vi "Teleop.vi"(10 "Match Info":T1={"Autonomous Elapsed Seconds"=0.0, "TeleOp Elapsed Seconds"=0.0, "Disabled Elapsed Seconds"=0.0, "Visited Autonomous"=FALSE, "Visited TeleOp"=FALSE, "Visited Disabled"=FALSE, "Autonomous Settings"={"Autonomous Style"=enum."Independent", "VI Refnum"=refnum}}, 11 "Call Context":T2) -> ()   [LabVIEW 2018]
doc: "This VI is called for each enabled TeleOp packet received from the DS. It is typically used to read from joysticks and other inputs and update I/O or setpoints for timed control loops. It should complete and return within 20 milliseconds or risk missing DS packets."
uses:
  <vilib>/Rock Robotics/WPI/DriverStation/WPI_DriverStationDerivedRobotMode.ctl
  <vilib>/Rock Robotics/WPI/DriverStation/WPI_DriverStationMatch Info.ctl
  <vilib>/Rock Robotics/WPI/Utilities/WPI_GetSetVariantRefNum.vi
  <vilib>/Rock Robotics/Network Tables/NT Write Boolean Array.vi
  <vilib>/Rock Robotics/Network Tables/NT Write Numeric Array.vi
  <vilib>/Rock Robotics/WPI/Ultrasonic/WPI_SonarMB1010AnalogRefNum Registry Get.vi
  <vilib>/Rock Robotics/WPI/Ultrasonic/WPI_SonarMB1010AnalogGetRange.vi
  Framework/Robot Global Data.vi
panel:
  out "Safe to drive Back (UnZucced)":bool
  out "Zucced?":bool
  in  "Sensor Margin of Error":dbl=2.0
  in  "Acceptable Hab Distance":dbl=12.0
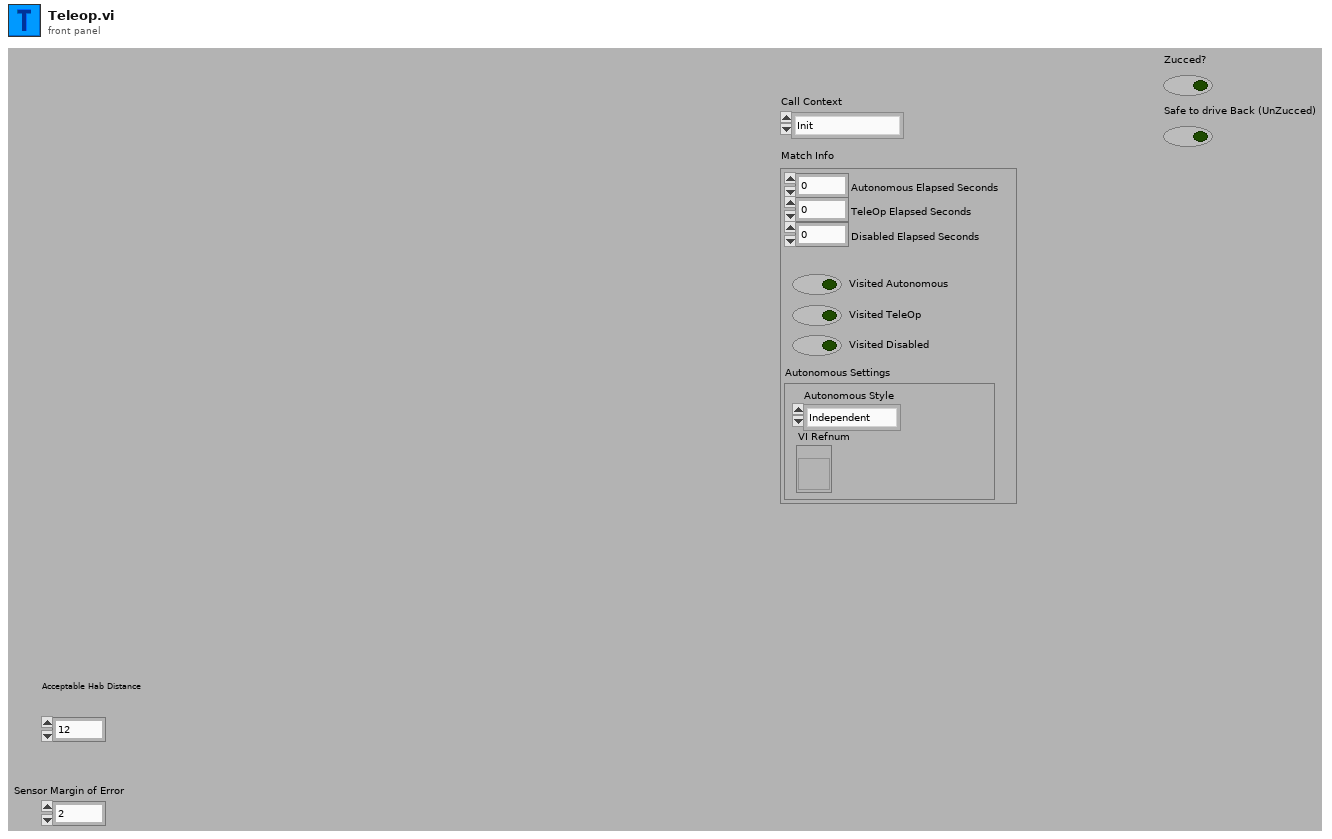
[diagram p1: front panel]
types:
  T1 = typedef "WPI_DriverStationMatch Info.ctl" = cluster{"Autonomous Elapsed Seconds":dbl, "TeleOp Elapsed Seconds":dbl, "Disabled Elapsed Seconds":dbl, "Visited Autonomous":bool, "Visited TeleOp":bool, "Visited Disabled":bool, "Autonomous Settings":cluster{"Autonomous Style":enum16{"Iterative", "Independent"}, "VI Refnum":refnum<vi>}}
  T2 = typedef "WPI_DriverStationDerivedRobotMode.ctl" = enum16{"Init", "Execute", "Stop"}
  T3 = typedef "WPI_JoystickDevRef.ctl" = cluster{"Device":T4}
  T4 = typedef "WPI_JoystickDeviceEnum.ctl" = enum16{"USB 0", "USB 1", "USB 2", "USB 3", "USB 4", "USB 5"}
  T5 = typedef "WPI_SonarMB1010AnalogDeviceRef.ctl" = cluster{"AIDeviceRef":T6, "Scaling factor (V/in)":dbl, "Average Bits":u8}
  T6 = typedef "WPI_AnalogChannelDevRef.ctl" = cluster{"DevStatus":errorcluster, "Analog Channel":T7}
  T7 = typedef "FPGA_AIChannel.ctl" = enum8{"AI 0", "AI 1", "AI 2", "AI 3", "AI MXP 0", "AI MXP 1", "AI MXP 2", "AI MXP 3", "Invalid"}
  T8 = typedef "WPI_ServoDeviceRef.ctl" = cluster{"DeviceStatus":errorcluster, "PWM Channel":T9, "DeadBand":T10}
  T9 = typedef "FPGA_DIOPWMChannel.ctl" = enum8{"PWM 0", "PWM 1", "PWM 2", "PWM 3", "PWM 4", "PWM 5", "PWM 6", "PWM 7", "PWM 8", "PWM 9", "PWM MXP 0", "PWM MXP 1", "PWM MXP 2", "PWM MXP 3", "PWM MXP 4", "PWM MXP 5", "PWM MXP 6", "PWM MXP 7", "PWM MXP 8", "PWM MXP 9", "Invalid"}
  T10 = typedef "WPI_PWMDeadband.ctl" = cluster{"Name":string, "maxPositivePwm":i32, "minPositivePwm":i32, "centerPwm":i32, "maxNegativePwm":i32, "minNegativePwm":i32, "angularRange":u16}
  T11 = typedef "WPI_MotorControlDeviceRef.ctl" = cluster{"DeviceStatus":errorcluster, "Type":T12, "PWM":cluster{"PWM Channel":T9, "DeadBand":T10}, "CAN":cluster{"Device Number":u8, "SetOutput VI Ref":variant, "GetOutput VI Ref":variant, "Enable VI Ref":variant, "Disable VI Ref":variant, "Data":variant}, "Invert":bool, "DIO PWM":cluster{"PWM \"Enable\" Channel":T9, "DIOChannel":T13, "PWM Rate":dbl}}
  T12 = typedef "WPI_MotorControlType.ctl" = enum16{"PWM", "CAN", "DIO PWM"}
  T13 = typedef "FPGA_DIOChannel.ctl" = enum8{"DIO 0", "DIO 1", "DIO 2", "DIO 3", "DIO 4", "DIO 5", "DIO 6", "DIO 7", "DIO 8", "DIO 9", "DIO MXP 0", "DIO MXP 1", "DIO MXP 2", "DIO MXP 3", "DIO MXP 4", "DIO MXP 5", "DIO MXP 6", "DIO MXP 7", "DIO MXP 8", "DIO MXP 9", "DIO MXP 10", "DIO MXP 11", "DIO MXP 12", "DIO MXP 13", "DIO MXP 14", "DIO MXP 15", "SPI Port CS1", "SPI Port CS2", "SPI Port CS3", "SPI Port MISO", "SPI Port MOSI", "Invalid"}
  T14 = typedef "WPI_DigitalOutputDevRef.ctl" = cluster{"DIO Channel":T13, "DevStatus":errorcluster}
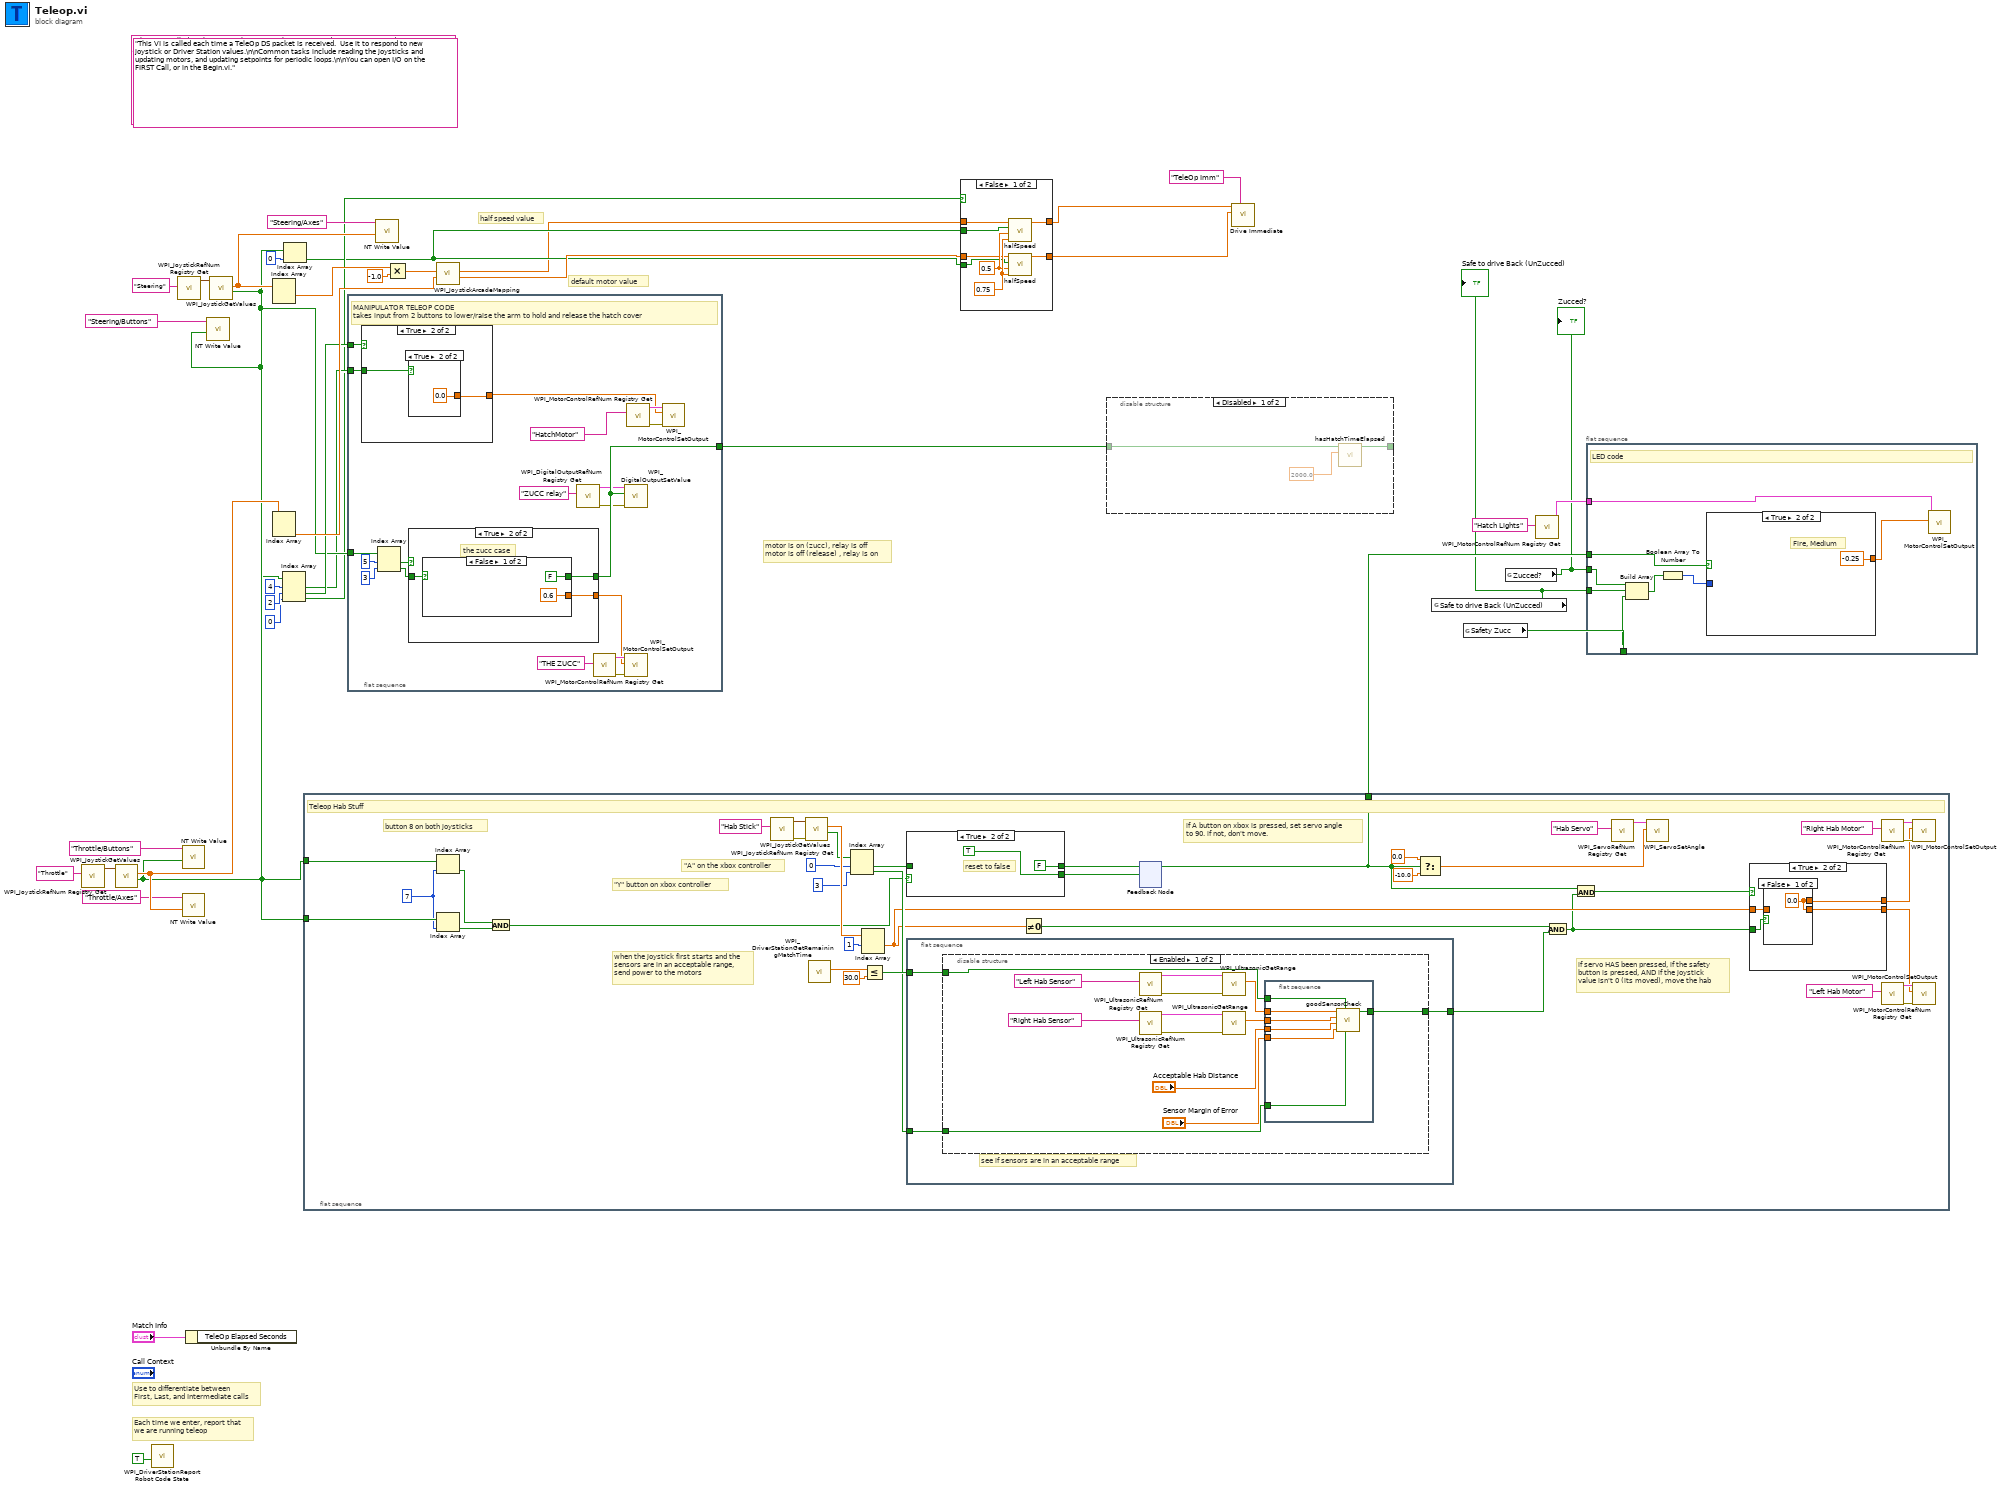
[diagram p0: block diagram]
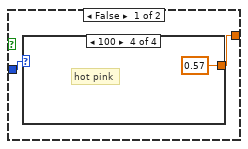
[diagram p4: hidden frame]
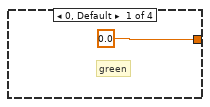
[diagram p5: hidden frame]
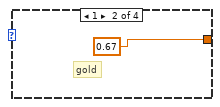
[diagram p6: hidden frame]
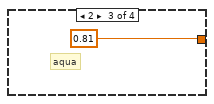
[diagram p7: hidden frame]
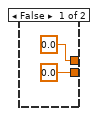
[diagram p9: hidden frame]
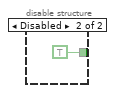
[diagram p11: hidden frame]
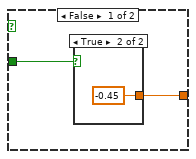
[diagram p12: hidden frame]
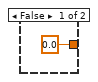
[diagram p13: hidden frame]
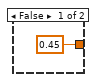
[diagram p14: hidden frame]
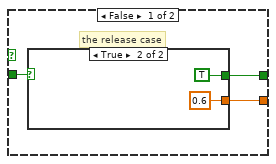
[diagram p15: hidden frame]
diagram:
  (unwired) "This VI is called each time a TeleOp DS packet is received.  Use it to respond to new joystick or Driver Station values.\n\nCommon tasks include reading the joysticks and updating motors, and updating setpoints for periodic loops.\n\nYou can open I/O on the FIRST Call, or in the Begin.vi."
  (unwired) "This VI is called each time a TeleOp DS packet is received.  Use it to respond to new joystick or Driver Station values.\n\nCommon tasks include reading the joysticks and updating motors, and updating setpoints for periodic loops.\n\nYou can open I/O on the FIRST Call, or in the Begin.vi."
  # "default motor value"
  # "half speed value"
  # "motor is on (zucc), relay is off\nmotor is off (release) , relay is on"
  # "Each time we enter, report that\nwe are running teleop"
  # "Use to differentiate between\nFirst, Last, and Intermediate calls"
  n1 = call <vilib>:"WPI_JoystickRefNum Registry Get.vi"("refnum name"="Throttle") -> ("JoystickDevRef"=w35:T3)  [unwired: 1 in, 9 out]
  n2 = call <vilib>:"WPI_JoystickGetValues.vi"("JoystickDevRef"=w35) -> ("Buttons"=w8:bool[], "Axes"=w31:dbl[])  [unwired: 6 in, 3 out]
  n3 = call <vilib>:"WPI_DriverStationReport Robot Code State.vi"("TeleOp"=TRUE ("Autonomous")) -> ()  [unwired: 10 in, 1 out]
  n4 = call <vilib>:"WPI_JoystickRefNum Registry Get.vi"("refnum name"="Steering") -> ("JoystickDevRef"=w29:T3)  [unwired: 1 in, 9 out]
  n5 = call-poly <vilib>:"NT Write Value.vi"("Boolean Array"=w8, "Name"="Throttle/Buttons") -> ()  [unwired: 9 in, 1 out]
  n6 = call-poly <vilib>:"NT Write Value.vi"("Numeric Array"=w31, "Name"="Throttle/Axes") -> ()  [unwired: 9 in, 1 out]
  n7 = Unbundle By Name("Match Info") -> ()  [unwired: 1 out]
  n8 = call <vilib>:"WPI_JoystickGetValues.vi"("JoystickDevRef"=w29) -> ("Buttons"=w17:bool[], "Axes"=w27:dbl[])  [unwired: 6 in, 3 out]
  n9 = call-poly <vilib>:"NT Write Value.vi"("Boolean Array"=w17, "Name"="Steering/Buttons") -> ()  [unwired: 9 in, 1 out]
  n10 = Index Array(array=w27) -> (element #1=w24:dbl)  [unwired: 2 in, 1 out]
  n11 = Index Array(array=w31) -> (element #2=w33:dbl)  [unwired: 2 in, 1 out]
  n12 = Index Array(array=w8, index #1=4 ("index"), index #2=2 ("index"), index #3=0 ("index")) -> (element #1=w12:bool, element #2=w18:bool, element #3=w6:bool)
  n13 = Index Array(array=w17, index=0) -> (element=w4:bool)
  n14 = flat-sequence {
    tunnel: w17 -> [w46]
    tunnel: w8 -> [w47]
    tunnel: [w41] -> w14
    frame #0 {
      w45 = 7 ("index")
      # "button 8 on both joysticks"
      # "if servo HAS been pressed, if the safety\nbutton is pressed, AND if the joystick\nvalue isn't 0 (its moved), move the hab"
      # "if A button on xbox is pressed, set servo angle\nto 90. if not, don't move."
      # "\"A\" on the xbox controller"
      # "\"Y\" button on xbox controller"
      # "when the joystick first starts and the\nsensors are in an acceptable range,\nsend power to the motors"
      # "Teleop Hab Stuff"
      n15 = Index Array(array=w47, index=w45) -> (element=w44:bool)
      n16 = Index Array(array=w46, index=w45) -> (element=w43:bool)
      n17 = And(x=w44, y=w43) -> (x .and. y?=w42:bool)
      n18 = call <vilib>:"WPI_JoystickRefNum Registry Get.vi"("refnum name"="Hab Stick") -> ("error out"=w76:errorcluster, "JoystickDevRef"=w75:T3)  [unwired: 9 in]
      n19 = call <vilib>:"WPI_JoystickGetValues.vi"("error in (no error)"=w76, "JoystickDevRef"=w75) -> ("Buttons"=w68:bool[], "Axes"=w74:dbl[])  [unwired: 5 in, 3 out]
      n20 = call <vilib>:"WPI_DriverStationGetRemainingMatchTime.vi"() -> ("Match Time(s)"=w78:sgl)  [unwired: 10 in, 1 out]
      n21 = Index Array(array=w68, index #1=0 ("index"), index #2=3 ("index")) -> (element #1=w49:bool, element #2=w65:bool)
      n22 = Index Array(array=w74, index #1=1 ("index")) -> (element #1=w61:dbl)  [unwired: 1 in, 1 out]
      n23 = Less Or Equal?(x=w78, y=sgl 30.0) -> (x <= y?=w69:bool)
      n24 = case shown="True" w42 {
        tunnel: [w79 FALSE] -> w50
        tunnel: w49 -> [w79 _]
        tunnel: [w79 TRUE] -> w48
        frame False {
        }
        frame True {
          # "reset to false"
        }
      }
      n25 = flat-sequence {
        tunnel: [w92] -> w70
        tunnel: w69 -> [w91]
        tunnel: w65 -> [w90]
        frame #0 {
          # "see if sensors are in an acceptable range"
          n26 = disable-structure shown="Enabled" {
            disable-tunnel: [w95 TRUE ("In range")] -> w92
            disable-tunnel: w91 -> [w94 _]
            disable-tunnel: w90 -> [w93 _]
            frame Enabled {
              n27 = call-poly <vilib>:"WPI_UltrasonicRefNum Registry Get.vi"("refnum name"="Left Hab Sensor") -> ("error out"=w100:errorcluster, "SonarMB1010AnalogDevRef"=w101:T5)  [unwired: 9 in]
              n28 = call-poly <vilib>:"WPI_UltrasonicRefNum Registry Get.vi"("refnum name"="Right Hab Sensor") -> ("error out"=w103:errorcluster, "SonarMB1010AnalogDevRef"=w104:T5)  [unwired: 9 in]
              n29 = call-poly <vilib>:"WPI_UltrasonicGetRange.vi"("error in"=w100, "SonarMB1010AnalogDevRef"=w101) -> ("Distance"=w96:dbl)  [unwired: 7 in, 2 out]
              n30 = call-poly <vilib>:"WPI_UltrasonicGetRange.vi"("error in"=w103, "SonarMB1010AnalogDevRef"=w104) -> ("Distance"=w97:dbl)  [unwired: 7 in, 2 out]
              n31 = flat-sequence {
                tunnel: "Acceptable Hab Distance" -> [w110]
                tunnel: "Sensor Margin of Error" -> [w109]
                tunnel: w97 -> [w111]
                tunnel: w96 -> [w112]
                tunnel: [w106] -> w95
                tunnel: w94 -> [w107]
                tunnel: w93 -> [w108]
                frame #0 {
                  n32 = call "goodSensorCheck.vi"("Temp Button Press"=w108, "Endgame yet?"=w107, "Sensor Margin of Error"=w109, "Acceptable Distance"=w110, "Right Sensor Value"=w111, "Left Sensor Value"=w112) -> ("In range"=w106:bool)  [unwired: 5 in]
                }
              }
            }
            frame Disabled {
            }
          }
        }
      }
      n33 = Not Equal To 0?(x=w61) -> (x != 0?=w72:bool)
      n34 = feedback #1() -> (w41:bool)  [unwired: 1 in]
      n35 = feedback-in #1(w50, w48) -> ()
      n36 = Select(t=0.0, s=w41, f=-10.0) -> (s? t:f=w62:dbl)
      n37 = And(x=w72, y=w70) -> (x .and. y?=w60:bool)
      n38 = And(x=w41, y=w60) -> (x .and. y?=w59:bool)
      n39 = call <vilib>:"WPI_ServoRefNum Registry Get.vi"("refnum name"="Hab Servo") -> ("ServoDeviceRef"=w40:T8)  [unwired: 9 in, 1 out]
      n40 = call <vilib>:"WPI_ServoSetAngle.vi"("Angle"=w62, "ServoDeviceRef"=w40) -> ()  [unwired: 8 in, 2 out]
      n41 = case shown="True" w59 {
        tunnel: w60 -> [_ w87]
        tunnel: w61 -> [_ w86]
        tunnel: [0.0 ("upper limit") w85] -> w55
        tunnel: [0.0 ("upper limit") w84] -> w51
        frame False {
        }
        frame True {
          n42 = case shown="False" w87 {
            tunnel: w86 -> [_ w89]
            tunnel: [w88 w89] -> w85
            tunnel: [w88 w89] -> w84
            frame False {
              w88 = 0.0 ("upper limit")
            }
            frame True {
            }
          }
        }
      }
      n43 = call <vilib>:"WPI_MotorControlRefNum Registry Get.vi"("refnum name"="Right Hab Motor") -> ("error out"=w58:errorcluster, "MotorControlDevRef"=w57:T11)  [unwired: 9 in]
      n44 = call <vilib>:"WPI_MotorControlRefNum Registry Get.vi"("refnum name"="Left Hab Motor") -> ("error out"=w53:errorcluster, "MotorControlDevRef"=w54:T11)  [unwired: 9 in]
      n45 = call <vilib>:"WPI_MotorControlSetOutput.vi"("error in (no error)"=w58, "Output"=w55, "MotorControlDevRef"=w57) -> ()  [unwired: 6 in, 3 out]
      n46 = call <vilib>:"WPI_MotorControlSetOutput.vi"("error in (no error)"=w53, "Output"=w51, "MotorControlDevRef"=w54) -> ()  [unwired: 6 in, 3 out]
    }
  }
  n47 = flat-sequence {
    tunnel: w17 -> [w132]
    tunnel: w18 -> [w131]
    tunnel: w12 -> [w130]
    tunnel: [w129] -> w16
    frame #0 {
      # "MANIPULATOR TELEOP CODE\ntakes input from 2 buttons to lower/raise the arm to hold and release the hatch cover"
      n48 = case shown="True" w131 {
        tunnel: [w134 w138] -> w114
        tunnel: w130 -> [w133 w137]
        frame False {
          n49 = case shown="True" w133 {
            tunnel: [0.0 -0.45] -> w134
            frame False {
            }
            frame True {
            }
          }
        }
        frame True {
          n50 = case shown="True" w137 {
            tunnel: [0.45 0.0] -> w138
            frame False {
            }
            frame True {
            }
          }
        }
      }
      n51 = Index Array(array=w132, index #1=5 ("index"), index #2=3 ("index")) -> (element #1=w117:bool, element #2=w116:bool)
      n52 = case shown="True" w117 {
        tunnel: w116 -> [w143 w148]
        tunnel: [w142 w147] -> w115
        tunnel: [w141 w146] -> w129
        frame False {
          # "the release case"
          n53 = case shown="True" w143 {
            tunnel: [_ 0.6] -> w142
            tunnel: [_ TRUE] -> w141
            frame False {
              # "do nothing if nothing\nis pressed"
            }
            frame True {
            }
          }
        }
        frame True {
          # "the zucc case"
          n54 = case shown="False" w148 {
            tunnel: [0.6 _] -> w147
            tunnel: [FALSE _] -> w146
            frame False {
            }
            frame True {
              # "do nothing if both\nare pressed"
            }
          }
        }
      }
      n55 = call <vilib>:"WPI_DigitalOutputRefNum Registry Get.vi"("refnum name"="ZUCC relay") -> ("error out"=w121:errorcluster, "DigitalOutputDevRef"=w120:T14)  [unwired: 9 in]
      n56 = call <vilib>:"WPI_MotorControlRefNum Registry Get.vi"("refnum name"="THE ZUCC") -> ("error out"=w124:errorcluster, "MotorControlDevRef"=w123:T11)  [unwired: 9 in]
      n57 = call <vilib>:"WPI_DigitalOutputSetValue.vi"("error in (no error)"=w121, "Value"=w129, "DigitalOutputDevRef"=w120) -> ()  [unwired: 7 in, 2 out]
      n58 = call <vilib>:"WPI_MotorControlSetOutput.vi"("error in (no error)"=w124, "Output"=w115, "MotorControlDevRef"=w123) -> ()  [unwired: 6 in, 3 out]
      n59 = call <vilib>:"WPI_MotorControlRefNum Registry Get.vi"("refnum name"="HatchMotor") -> ("error out"=w127:errorcluster, "MotorControlDevRef"=w126:T11)  [unwired: 9 in]
      n60 = call <vilib>:"WPI_MotorControlSetOutput.vi"("error in (no error)"=w127, "Output"=w114, "MotorControlDevRef"=w126) -> ()  [unwired: 6 in, 3 out]
    }
  }
  n61 = call-poly <vilib>:"NT Write Value.vi"("Numeric Array"=w27, "Name"="Steering/Axes") -> ()  [unwired: 9 in, 1 out]
  n62 = Multiply(x=w24, y=-1.0) -> (x*y=w23:dbl)
  n63 = call <vilib>:"WPI_JoystickArcadeMapping.vi"("Y axis value"=w33, "X axis value"=w23) -> ("Right Motor Value"=w5:dbl, "Left Motor Value"=w3:dbl)  [unwired: 8 in]
  n64 = case shown="False" w6 {
    tunnel: w4 -> [w156 _]
    tunnel: w5 -> [w155 w159]
    tunnel: w4 -> [w154 _]
    tunnel: w3 -> [w153 w160]
    tunnel: [w152 w159] -> w2
    tunnel: [w151 w160] -> w1
    frame False {
      w158 = 0.75 ("Default Power")
      w157 = 0.5 ("Fraction")
      n65 = call "halfSpeed"("Default Power"=w158, "Fraction"=w157, "Slow speed?"=w154, "Motor Input"=w153) -> ("Motor Output"=w151:dbl)  [unwired: 7 in]
      n66 = call "halfSpeed"("Default Power"=w158, "Fraction"=w157, "Slow speed?"=w156, "Motor Input"=w155) -> ("Motor Output"=w152:dbl)  [unwired: 7 in]
    }
    frame True {
    }
  }
  n67 = disable-structure shown="Disabled" {
    disable-tunnel: w16 -> [w163 _]
    disable-tunnel: [w162 _] -> _
    frame Disabled {
      n68 = call "hasHatchTimeElapsed"("valve wait time"=2000.0, "Valve button pressed?"=w163) -> ("Valve good to release?"=w162:bool)  [unwired: 9 in]
    }
    frame Enabled {
    }
  }
  n69 = call "Drive Immediate.vi"("Description"="TeleOp Imm", "Right Setpoint"=w2, "Left Setpoint"=w1) -> ()  [unwired: 8 in, 1 out]
  n70 = global read "Robot Global Data.vi" "Safe to drive Back (UnZucced)"() -> (w10:bool)
  "Safe to drive Back (UnZucced)" <- w10
  n71 = global read "Robot Global Data.vi" "Safety Zucc"() -> (w9:bool)
  n72 = global read "Robot Global Data.vi" "Zucced?"() -> (w11:bool)
  "Zucced?" <- w11
  n73 = call <vilib>:"WPI_MotorControlRefNum Registry Get.vi"("refnum name"="Hatch Lights") -> ("MotorControlDevRef"=w13:T11)  [unwired: 9 in, 1 out]
  n74 = flat-sequence {
    tunnel: w14 -> [w164]
    tunnel: w13 -> [w169]
    tunnel: w11 -> [w168]
    tunnel: w10 -> [w167]
    tunnel: w9 -> [w165]
    frame #0 {
      # "LED code"
      n75 = Build Array(w168, w167, w165) -> (w171:bool[])
      n76 = Boolean Array To Number(Boolean array=w171) -> (number=w170:u32)
      n77 = case shown="True" w164 {
        tunnel: w170 -> [w173 _]
        tunnel: [w172 -0.25] -> w166
        frame False {
          n78 = case shown="100" w173 {
            tunnel: [0.0 0.67 0.81 0.57] -> w172
            frame 0, Default {
              # "green"
            }
            frame 1 {
              # "gold"
            }
            frame 2 {
              # "aqua"
            }
            frame 4 {
              # "hot pink"
            }
          }
        }
        frame True {
          # "Fire, Medium"
        }
      }
      n79 = call <vilib>:"WPI_MotorControlSetOutput.vi"("Output"=w166, "MotorControlDevRef"=w169) -> ()  [unwired: 7 in, 3 out]
    }
  }
